vi "RT main 2 local variable.vi"() -> ()   [LabVIEW 2017]
doc: "This example demonstrates how to acquire a continuous amount of data (Waveform) using the DAQ device's internal clock. It also shows how to synchronize two devices for different device families (E Series, S Series, M Series, X Series, DSA, and SC Express), to simultaneously acquire the data.\n\nFor instructions on how to connect your signals to the DAQ device, refer to your device documentation."
uses:
  typedefs/Data.ctl
  <vilib>/Utility/RT CPU Load.ctl
  <vilib>/Utility/error.llb/DialogType.ctl
  <vilib>/DAQmx/read.llb/DAQmx Read (Analog 1D Wfm NChan NSamp).vi
  <vilib>/Analysis/baseanly.llb/Mean (DBL).vi
  <vilib>/DAQmx/read.llb/DAQmx Read (Analog Wfm 1Chan NSamp).vi
  <vilib>/Analysis/5stat.llb/RMS (DBL).vi
  <vilib>/DAQmx/read.llb/DAQmx Read (Analog DBL 1Chan 1Samp).vi
  <vilib>/DAQmx/create/channels.llb/DAQmx Create Channel (AI-Voltage-Basic).vi
  <vilib>/DAQmx/create/channels.llb/DAQmx Create Channel (AI-Temperature-Thermocouple).vi
  <vilib>/DAQmx/configure/timing.llb/DAQmx Timing (Sample Clock).vi
  <vilib>/httpClient/POSTBuffer.vi
  <vilib>/DAQmx/miscellaneous.llb/DAQmx Fill In Error Info.vi
  <vilib>/Analysis/NI_AALBase.lvlib
  <vilib>/httpClient/LabVIEWHTTPClient.lvlib
  <vilib>/NI_Real-Time Target Support.lvlib
  <vilib>/Analysis/NI_AALPro.lvlib
panel:
  out "output cluster":T1={"RMS"=0.00029761559443340104, "RPM"=4.976174049057853, "Voltage"=24.13586620003172, "Current"=-0.01197022918749992, "Temperature"=22.47037779695891} {"RMS" format="%0.6f"; "RPM" format="%0.2f"; "Voltage" format="%0.2f"; "Current" format="%0.2f"; "Temperature" format="%0.2f"}
  in  "Ipad 1":bool
  in  "Ipad 3":bool
  in  "Ipad 2":bool
  in  "Button 3":bool
  in  "Button 2":bool
  in  "Buttoon 1":bool
  in  "String":string="http://10.156.1.111:8001/cRioWebservice/weURL"
  in  "Tab Control":enum32{"Main", "Setup   ", "Debug"}(tab)=enum."Setup   "
  out "Output States":bool[](array[boolean])
  out "From Thingworx":bool[](array[boolean])
  out "Voltage":dbl(graph)=22.47037779695891 caption="Thermocouple waveform"
  out "Current":dbl(graph)=22.47037779695891 caption="Thermocouple waveform"
  out "RPM":dbl(graph)=22.47037779695891 caption="Thermocouple waveform"
  out "Temperature":dbl(graph)=22.47037779695891 caption="Thermocouple waveform"
  out "Vibration":waveform(dbl)(graph)={"t0"=timestamp(3612407740.6938596 s since 1904-01-01), "dt"=3.906249999999998e-05, "Y"=[], "attributes"=variant("NI_ChannelName"=variant(string "Mod1/ai0"), "NI_UnitDescription"=variant(string "Volts"))}
  out "Data":T2
  out "Buttons":bool[](array[boolean])
  in  "stop":bool
  in  "Vibration Sample":i32=25600
  in  "9234 Sample Rate":dbl=25600.0
  in  "9234 Channel":tag="Mod1/ai0"
  in  "9201 Samples to Read":i32=25600
  in  "9201 Sample Rate":dbl=25600.0
  in  "9201 Channel":tag="Mod3/ai0:2"
  in  "CJC Channel":refnum<k21>
  in  "CJC Value":dbl=25.0 format="%0.2f"
  in  "CJC Source":i32(ring)=10116 items=["Built-In"=10200, "Constant Value"=10116, "Channel"=10113]
  in  "Thermocouple Type":i32(ring)=10073 items=["J"=10072, "K"=10073, "N"=10077, "R"=10082, "S"=10085, "T"=10086, "B"=10047, "E"=10055]
  in  "Units":i32(ring)=10143 items=["Deg C"=10143, "Deg F"=10144, "Kelvins"=10325, "Deg R"=10145, "From Custom Scale"=10065]
  in  "Max Temperature":dbl=35.0
  in  "Min Temperature":dbl=-30.0
  in  "Thermocouple Sample":i32=1
  in  "Thermocouple":tag="Mod2/ai0"
  in  "Voltage correction factor":dbl=5.0
  in  "Current correction factor":dbl=10.0
  in  "Thingworx Key":string="1ec2abed-8590-4b69-8e20-7ebb8ff4261c"
  in  "ThingWorx URL":string="http://10.156.1.88:8080/Thingworx/Things/NIMotor/Services/ReceiveData?postParameter=json"
  out "CPU loads":T3[](array[typedef])=[{"Total (%)"=49.32460172385931, "Time Critical (%)"=0.3247606240343923, "Timed Structures (%)"=0.0, "High (%)"=0.0, "Above Normal (%)"=0.0, "Normal (%)"=48.388661684659795, "Background (%)"=0.0, "Idle (%)"=50.67539827614069, "ISR (%)"=0.6111794151651194}, {"Total (%)"=40.05228188925075, "Time Critical (%)"=0.0, "Timed Structures (%)"=0.0, "High (%)"=0.0, "Above Normal (%)"=0.0, "Normal (%)"=39.81026940927922, "Background (%)"=0.0, "Idle (%)"=59.94771811074925, "ISR (%)"=0.24201247997152983}] {"ISR (%)" format="%#.2f"; "Idle (%)" format="%#.2f"; "Background (%)" format="%#.2f"; "Normal (%)" format="%#.2f"; "Above Normal (%)" format="%#.2f"; "High (%)" format="%#.2g"; "Timed Structures (%)" format="%#.2g"; "Time Critical (%)" format="%#.2g"; "Total (%)" format="%#.2g"}
  out "Loop Count":i32=1197
  out "Loop Count 2":i32=1194
  out "Loop Count 3":i32=725
  out "JSON Output":string
  out "error out":errorcluster
  # "(Not Used)"
  # "Vibration"
  # "Motor Voltage"
  # "Motor Current"
  # "RPM"
  # "Temperature"
  # "Thingworx Setup"
  # "9234 Settings"
  # "9201 Settings"
  # "9211 Settings"
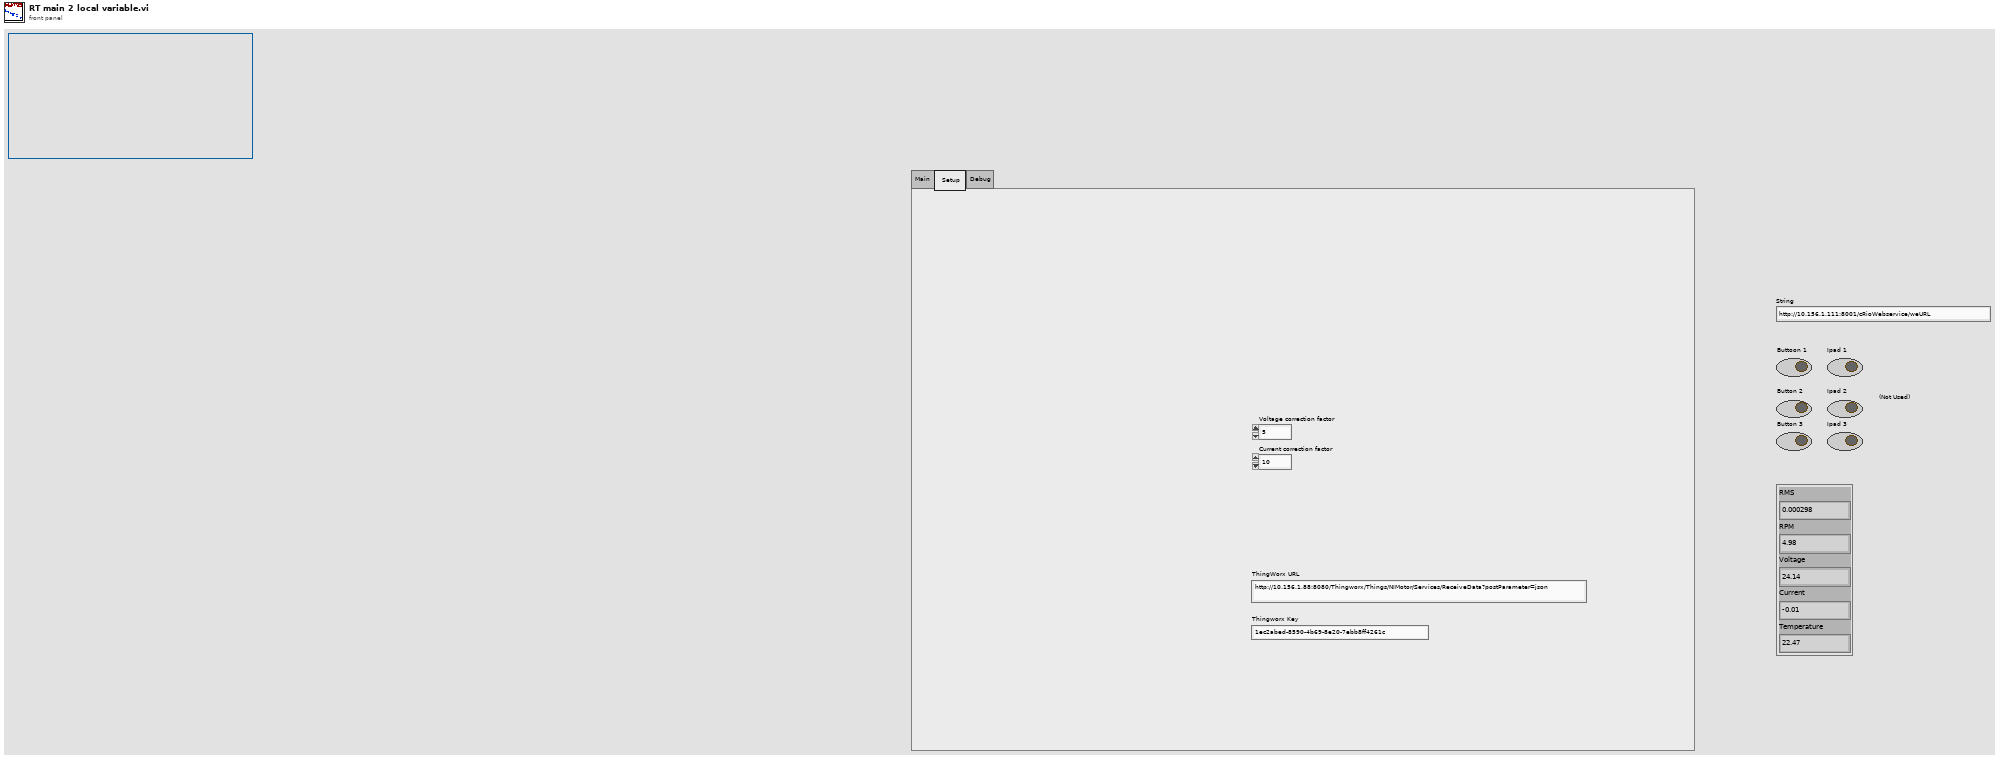
[diagram p1: front panel]
types:
  T1 = typedef "Data.ctl" = cluster{"RMS":dbl, "RPM":dbl, "Voltage":dbl, "Current":dbl, "Temperature":dbl}
  T2 = cluster{"RMS":dbl, "RPM":dbl, "Voltage":dbl, "Current":dbl, "Temperature":dbl}
  T3 = typedef "NI_Real-Time Target Support.lvlib/RT CPU Load.ctl" = cluster{"Total (%)":dbl, "Time Critical (%)":dbl, "Timed Structures (%)":dbl, "High (%)":dbl, "Above Normal (%)":dbl, "Normal (%)":dbl, "Background (%)":dbl, "Idle (%)":dbl, "ISR (%)":dbl}
  T4 = typedef "DialogType.ctl" = u16
  T5 = typedef "LabVIEWHTTPClient.lvlib/ClientHandle.ctl" = refnum<k1>
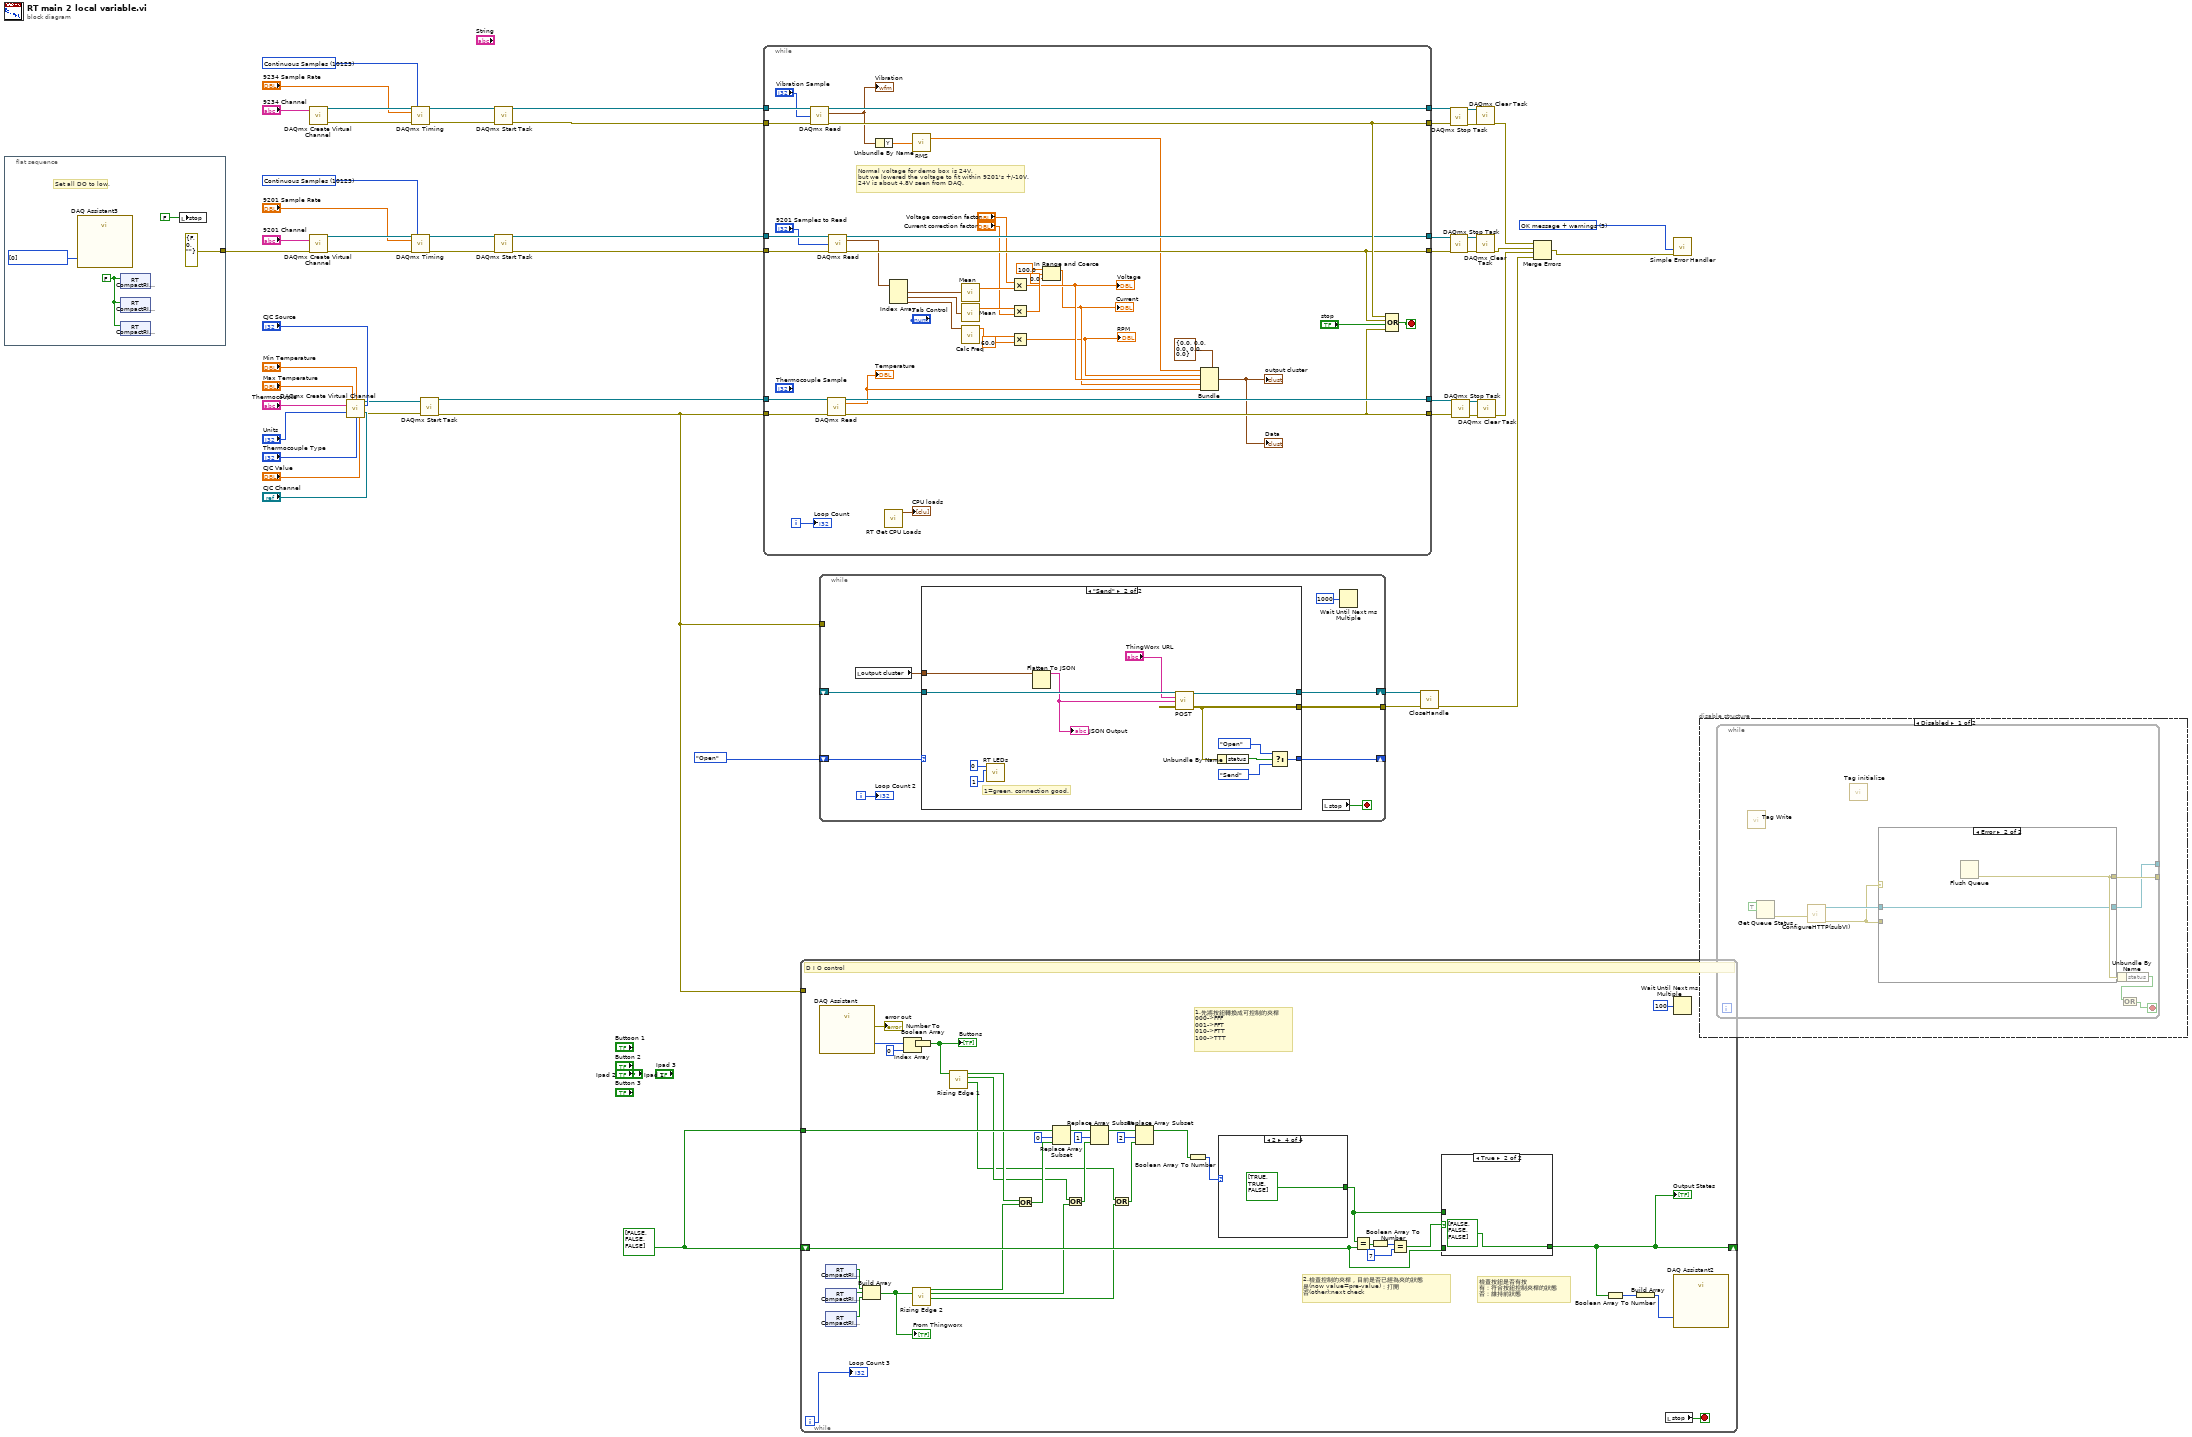
[diagram p0: block diagram]
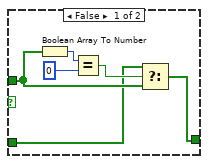
[diagram p2: hidden frame]
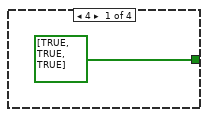
[diagram p3: hidden frame]
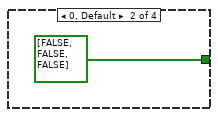
[diagram p4: hidden frame]
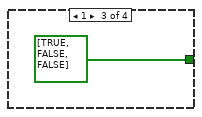
[diagram p5: hidden frame]
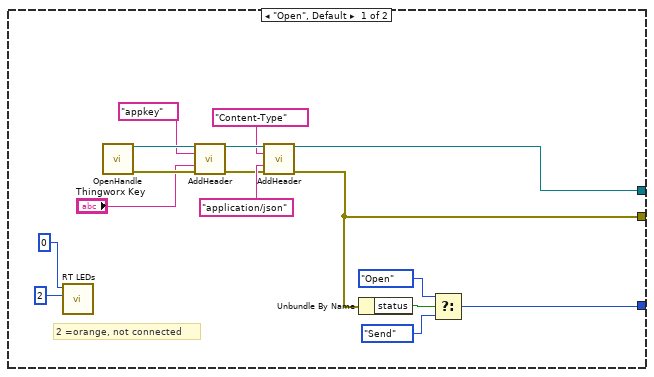
[diagram p6: hidden frame]
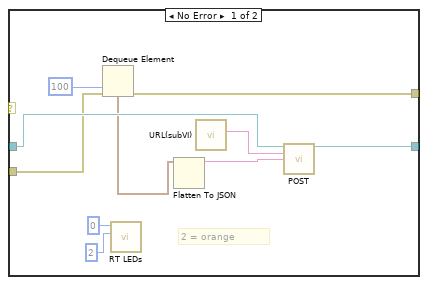
[diagram p7: hidden frame]
diagram:
  w5 = bool[] [FALSE, FALSE, FALSE]
  w10 = 10123 items=["Finite Samples"=10178, "Continuous Samples"=10123, "Hardware Timed Single Point"=12522] ("sample mode")
  w11 = 10123 items=["Finite Samples"=10178, "Continuous Samples"=10123, "Hardware Timed Single Point"=12522] ("sample mode")
  w30 = T4 3 items=["no dialog", "OK message", "continue or stop message", "OK message + warnings", "continue/stop + warnings"] ("type of dialog (OK msg:1)")
  n1 = flat-sequence {
    tunnel: [errorcluster {"status"=FALSE, "code"=0, "source"=""} ("error in")] -> w2
    frame #0 {
      w54 = FALSE ("X")
      # "Set all DO to low."
      n2 = call "DAQ Assistant3"("data"=u32[] [0]) -> ()  [unwired: 17 in, 2 out]
      n3 = shared-variable "RT CompactRIO Target \\variable.lvlib\\X"(w54) -> ()  [unwired: 1 in, 1 out]
      n4 = shared-variable "RT CompactRIO Target \\variable.lvlib\\Y"(w54) -> ()  [unwired: 1 in, 1 out]
      n5 = shared-variable "RT CompactRIO Target \\variable.lvlib\\Z"(w54) -> ()  [unwired: 1 in, 1 out]
      n6 = local write "stop"(FALSE ("Stop")) -> ()
    }
  }
  n7 = call-poly <vilib>:"DAQmx Create Virtual Channel.vi"("physical channels"="9234 Channel") -> ("task out"=w37:refnum<k21>, "error out"=w36:errorcluster)  [unwired: 13 in]
  n8 = call-poly <vilib>:"DAQmx Create Virtual Channel.vi"("physical channels"="9201 Channel", "error in"=w2) -> ("task out"=w33:refnum<k21>, "error out"=w35:errorcluster)  [unwired: 12 in]
  n9 = call-poly <vilib>:"DAQmx Create Virtual Channel.vi"("maximum value"="Max Temperature", "minimum value"="Min Temperature", "physical channels"="Thermocouple", "cjc source"="CJC Source", "units"="Units", "cjc channel"="CJC Channel", "thermocouple type"="Thermocouple Type", "cjc value"="CJC Value") -> ("task out"=w13:refnum<k21>, "error out"=w9:errorcluster)  [unwired: 6 in]
  n10 = call-poly <vilib>:"DAQmx Timing.vi"("task/channels in"=w37, "sample mode"=w10, "rate"="9234 Sample Rate", "error in"=w36) -> ("task out"=w12:refnum<k21>, "error out"=w28:errorcluster)  [unwired: 10 in]
  n11 = call-poly <vilib>:"DAQmx Timing.vi"("task/channels in"=w33, "sample mode"=w11, "rate"="9201 Sample Rate", "error in"=w35) -> ("task out"=w34:refnum<k21>, "error out"=w32:errorcluster)  [unwired: 10 in]
  n12 = call <vilib>:"DAQmx Start Task.vi"("task/channels in"=w13, "error in"=w9) -> ("task out"=w27:refnum<k21>, "error out"=w1:errorcluster)  [unwired: 12 in]
  n13 = call <vilib>:"DAQmx Start Task.vi"("task/channels in"=w12, "error in"=w28) -> ("task out"=w53:refnum<k21>, "error out"=w52:errorcluster)  [unwired: 12 in]
  n14 = call <vilib>:"DAQmx Start Task.vi"("task/channels in"=w34, "error in"=w32) -> ("task out"=w51:refnum<k21>, "error out"=w50:errorcluster)  [unwired: 12 in]
  n15 = while {
    tunnel: w27 -> [w89]
    tunnel: w1 -> [w88]
    tunnel: [w87] -> w24
    tunnel: [w86] -> w23
    tunnel: w53 -> [w96]
    tunnel: [w80] -> w49
    tunnel: w51 -> [w93]
    tunnel: [w81] -> w45
    tunnel: w50 -> [w92]
    tunnel: [w91] -> w44
    tunnel: w52 -> [w95]
    tunnel: [w94] -> w48
    i -> [w79]
    stop <- w97 stop-if-true
    # "Normal voltage for demo box is 24V,\nbut we lowered the voltage to fit within 9201's +/-10V.\n24V is about 4.8V seen from DAQ."
    n16 = call-poly <vilib>:"DAQmx Read.vi"("task/channels in"=w96, "number of samples per channel"="Vibration Sample", "error in"=w95) -> ("task out"=w80:refnum<k21>, "data"=w77:waveform(dbl), "error out"=w94:errorcluster)  [unwired: 10 in]
    "Vibration" <- w77
    n17 = call-poly <vilib>:"DAQmx Read.vi"("task/channels in"=w89, "error in"=w88) -> ("task out"=w87:refnum<k21>, "data"=w83:dbl, "error out"=w86:errorcluster)  [unwired: 11 in]
    "Temperature" <- w83
    n18 = call-poly <vilib>:"DAQmx Read.vi"("task/channels in"=w93, "number of samples per channel"="9201 Samples to Read", "error in"=w92) -> ("task out"=w81:refnum<k21>, "data"=w73:waveform(dbl)[], "error out"=w91:errorcluster)  [unwired: 10 in]
    n19 = Unbundle By Name(w77) -> ("Y"=w76:dbl[])
    n20 = call <vilib>:"RT Get CPU Loads.vi"() -> ("CPU loads"=→"CPU loads":T3[])  [unwired: 10 in, 1 out]
    n21 = Index Array(array=w73) -> (element #1=w84:waveform(dbl), element #2=w82:waveform(dbl), element #3=w68:waveform(dbl))  [unwired: 3 in]
    n22 = call-poly <vilib>:"RMS.vi"("X"=w76) -> ("rms value"=w75:dbl)  [unwired: 1 out]
    n23 = call-poly <vilib>:"Mean.vi"("X"=w82) -> ("mean"=w70:dbl)  [unwired: 1 out]
    n24 = call "Calc Freq.vi"("waveform"=w68) -> ("Freq"=w67:dbl)  [unwired: 10 in]
    n25 = call-poly <vilib>:"Mean.vi"("X"=w84) -> ("mean"=w72:dbl)  [unwired: 1 out]
    n26 = Multiply(x="Voltage correction factor", y=w72) -> (x*y=w62:dbl)
    "Voltage" <- w62
    n27 = Multiply(x=w70, y="Current correction factor") -> (x*y=w65:dbl)
    n28 = Multiply(x=w67, y=60.0) -> (x*y=w60:dbl)
    "RPM" <- w60
    n29 = In Range and Coerce(upper limit=100.0, x=w65, lower limit=0.0) -> (coerced(x)=w61:dbl)  [unwired: 1 out]
    "Current" <- w61
    n30 = Bundle(cluster=T1 {"RMS"=0.0, "RPM"=0.0, "Voltage"=0.0, "Current"=0.0, "Temperature"=0.0} ("Data"), "RMS"=w75, "RPM"=w60, "Voltage"=w62, "Current"=w61, "Temperature"=w83) -> (→"output cluster" →"Data":T1)
    n31 = Compound Arithmetic op=OR(w94, w91, "stop", w86) -> (w97:bool)
    "Loop Count" <- w79
  }
  n32 = while {
    shift-right: [w98] -> _
    shift-left: w5 -> [w119]
    tunnel: w5 -> [w118]
    tunnel: w1 -> [_]
    i -> [w110]
    stop <- w117 stop-if-true
    # "1.先將按鈕轉換成可控制的夾桿\n000->FFF\n001->FFT\n010->FTT\n100->TTT"
    # "檢查按鈕是否有按\n有：符合按鈕控制夾桿的狀態\n否：維持前狀態"
    # "2.檢查控制的夾桿，目前是否已經為夾的狀態\n是(now value=pre-value)：打開\n否(other):next check"
    # "D I O control"
    n33 = call "DAQ Assistant"() -> ("data"=w116:u32[], "error out"=→"error out":errorcluster)  [unwired: 17 in, 1 out]
    n34 = shared-variable "RT CompactRIO Target \\variable.lvlib\\X"() -> (w106:bool)  [unwired: 1 in, 1 out]
    n35 = shared-variable "RT CompactRIO Target \\variable.lvlib\\Y"() -> (w105:bool)  [unwired: 1 in, 1 out]
    n36 = shared-variable "RT CompactRIO Target \\variable.lvlib\\Z"() -> (w104:bool)  [unwired: 1 in, 1 out]
    n37 = Build Array(w106, w105, w104) -> (w99:bool[])
    "From Thingworx" <- w99
    n38 = Index Array(array=w116, index=0) -> (element=w114:u32)
    n39 = call "Rising Edge 2.vi"("Boolean Array"=w99) -> ("triggered? 3"=w101:bool, "triggered? 2"=w102:bool, "triggered? 1"=w103:bool)  [unwired: 8 in]
    n40 = Number To Boolean Array(number=w114) -> (Boolean array=w100:bool[])
    "Buttons" <- w100
    n41 = call "Rising Edge 1.vi"("Boolean Array"=w100) -> ("triggered? 3"=w111:bool, "triggered? 2"=w112:bool, "triggered? 1"=w113:bool)  [unwired: 8 in]
    n42 = Or(x=w113, y=w103) -> (x .or. y?=w129:bool)
    n43 = Replace Array Subset(array=w118, new element=w129, index=0) -> (w134:bool[])
    n44 = Or(x=w112, y=w102) -> (x .or. y?=w128:bool)
    n45 = Replace Array Subset(array=w134, new element=w128, index=1) -> (w133:bool[])
    n46 = Or(x=w111, y=w101) -> (x .or. y?=w127:bool)
    n47 = Replace Array Subset(array=w133, new element=w127, index=2) -> (w120:bool[])
    n48 = Boolean Array To Number(Boolean array=w120) -> (number=w122:u32)
    n49 = case shown="2" w122 {
      tunnel: [bool[] [TRUE, TRUE, TRUE] ("Button") bool[] [FALSE, FALSE, FALSE] ("Button") bool[] [TRUE, FALSE, FALSE] ("Button") bool[] [TRUE, TRUE, FALSE] ("Button")] -> w126
      frame 4 {
      }
      frame 0, Default {
      }
      frame 1 {
      }
      frame 2 {
      }
    }
    n50 = Equal?(x=w126, y=w119) -> (x = y?=w123:bool[])
    n51 = Boolean Array To Number(Boolean array=w123) -> (number=w124:u32)
    n52 = Equal?(x=w124, y=u32 7) -> (x = y?=w125:bool)
    n53 = case shown="True" w125 {
      tunnel: [w136 bool[] [FALSE, FALSE, FALSE] ("Button")] -> w98
      tunnel: w126 -> [w138 _]
      tunnel: w119 -> [w137 _]
      frame False {
        n54 = Boolean Array To Number(Boolean array=w138) -> (number=w140:u32)
        n55 = Equal?(x=w140, y=u32 0) -> (x = y?=w139:bool)
        n56 = Select(t=w137, s=w139, f=w138) -> (s? t:f=w136:bool[])
      }
      frame True {
      }
    }
    "Output States" <- w98
    n57 = Boolean Array To Number(Boolean array=w98) -> (number=w108:u32)
    n58 = Build Array(w108) -> (w107:u32[])
    n59 = local read "stop"() -> (w117:bool)
    n60 = Wait Until Next ms Multiple(millisecond multiple=u32 100) -> ()  [unwired: 1 out]
    n61 = call "DAQ Assistant2"("data"=w107) -> ()  [unwired: 17 in, 2 out]
    "Loop Count 3" <- w110
  }
  n62 = while {
    shift-right: [w154] -> _
    shift-left: enum16{"Open", "Send"}."Open" -> [w155]
    shift-right: [w153] -> w7
    shift-left: _ -> [w152]
    tunnel: [w150] -> w8
    tunnel: w1 -> [_]
    i -> [w149]
    stop <- w151 stop-if-true
    n63 = local read "output cluster"() -> (w147:T1)
    n64 = case shown="\"Send\"" w155 {
      tunnel: [w168 w182] -> w154
      tunnel: [w157 w178] -> w153
      tunnel: w152 -> [_ w179]
      tunnel: [w156 w174] -> w150
      tunnel: w147 -> [_ w173]
      frame "Open", Default {
        # "2 =orange, not connected"
        n65 = call <vilib>:"RT LEDs.vi"("State"=2, "LED Num"=0) -> ()  [unwired: 4 in, 2 out]
        n66 = call <vilib>:"OpenHandle.vi"() -> ("client handle out"=w165:T5, "error out"=w164:errorcluster)  [unwired: 14 in]
        n67 = call <vilib>:"AddHeader.vi"("client handle"=w165, "header"="appkey", "value"="Thingworx Key", "error in (no error)"=w164) -> ("client handle out"=w163:T5, "error out"=w160:errorcluster)  [unwired: 10 in]
        n68 = call <vilib>:"AddHeader.vi"("client handle"=w163, "header"="Content-Type", "value"="application/json", "error in (no error)"=w160) -> ("client handle out"=w157:T5, "error out"=w156:errorcluster)  [unwired: 10 in]
        n69 = Unbundle By Name(w156) -> ("status"=w171:bool)
        n70 = Select(t=enum16{"Open", "Send"}."Open", s=w171, f=enum16{"Open", "Send"}."Send") -> (s? t:f=w168:enum16{"Open", "Send"})
      }
      frame "Send" {
        # "1=green, connection good."
        n71 = call <vilib>:"RT LEDs.vi"("State"=1, "LED Num"=0) -> ()  [unwired: 4 in, 2 out]
        n72 = Flatten To JSON(anything=w173) -> (JSON string=w175:string)  [unwired: 2 in, 1 out]
        "JSON Output" <- w175
        n73 = call-poly <vilib>:"POST.vi"("client handle"=w179, "url"="ThingWorx URL", "buffer"=w175) -> ("client handle out"=w178:T5, "error out"=w174:errorcluster)  [unwired: 9 in, 2 out]
        n74 = Unbundle By Name(w174) -> ("status"=w183:bool)
        n75 = Select(t=enum16{"Open", "Send"}."Open", s=w183, f=enum16{"Open", "Send"}."Send") -> (s? t:f=w182:enum16{"Open", "Send"})
      }
    }
    n76 = local read "stop"() -> (w151:bool)
    n77 = Wait Until Next ms Multiple(millisecond multiple=u32 1000) -> ()  [unwired: 1 out]
    "Loop Count 2" <- w149
  }
  n78 = call <vilib>:"CloseHandle.vi"("client handle"=w7, "error in (no error)"=w8) -> ("error out"=w3:errorcluster)  [unwired: 13 in]
  n79 = call <vilib>:"DAQmx Stop Task.vi"("task/channels in"=w49, "error in"=w48) -> ("task out"=w46:refnum<k21>, "error out"=w47:errorcluster)  [unwired: 12 in]
  n80 = call <vilib>:"DAQmx Stop Task.vi"("task/channels in"=w45, "error in"=w44) -> ("task out"=w42:refnum<k21>, "error out"=w43:errorcluster)  [unwired: 12 in]
  n81 = call <vilib>:"DAQmx Stop Task.vi"("task/channels in"=w24, "error in"=w23) -> ("task out"=w26:refnum<k21>, "error out"=w25:errorcluster)  [unwired: 12 in]
  n82 = call <vilib>:"DAQmx Clear Task.vi"("task in"=w46, "error in"=w47) -> ("error out"=w41:errorcluster)  [unwired: 13 in]
  n83 = call <vilib>:"DAQmx Clear Task.vi"("task in"=w42, "error in"=w43) -> ("error out"=w40:errorcluster)  [unwired: 13 in]
  n84 = call <vilib>:"DAQmx Clear Task.vi"("task in"=w26, "error in"=w25) -> ("error out"=w22:errorcluster)  [unwired: 13 in]
  n85 = Merge Errors(w41, w40, w22, w3) -> (w4:errorcluster)
  n86 = call <vilib>:"Simple Error Handler.vi"("type of dialog (OK msg:1)"=w30, "error in (no error)"=w4) -> ()  [unwired: 3 in, 5 out]
  n87 = disable-structure shown="Disabled" {
    frame Disabled {
      n88 = while {
        tunnel: [w189] -> _
        tunnel: [w186] -> _
        stop <- w190 stop-if-true
        n89 = call "Tag Write.vi"() -> ()  [unwired: 19 in, 1 out]
        n90 = Get Queue Status(return elements? (F)=TRUE) -> (error out=w188:errorcluster)  [unwired: 2 in, 7 out]
        n91 = call "ConfigureHTTP(subVI).vi"("error in (no error)"=w188) -> ("error out"=w184:errorcluster, "Refnum out"=w187:T5)  [unwired: 9 in]
        n92 = call "Tag initialize.vi"() -> ()  [unwired: 14 in, 6 out]
        n93 = case shown="Error" w184 {
          tunnel: [w197 w203] -> w189
          tunnel: w187 -> [w199 w202]
          tunnel: [w198 w202] -> w186
          tunnel: w184 -> [w196 _]
          frame No Error {
            # "2 = orange"
            n94 = Dequeue Element(timeout in ms (-1)=100, error in (no error)=w196) -> (element=w194:T2, error out=w197:errorcluster)  [unwired: 1 in, 2 out]
            n95 = call <vilib>:"RT LEDs.vi"("State"=2, "LED Num"=0) -> ()  [unwired: 4 in, 2 out]
            n96 = Flatten To JSON(anything=w194) -> (JSON string=w195:string)  [unwired: 2 in, 1 out]
            n97 = call "URL(subVI).vi"() -> ("URL"=w200:string)  [unwired: 11 in]
            n98 = call-poly <vilib>:"POST.vi"("client handle"=w199, "url"=w200, "buffer"=w195) -> ("client handle out"=w198:T5)  [unwired: 9 in, 3 out]
          }
          frame Error {
            n99 = Flush Queue() -> (error out=w203:errorcluster)  [unwired: 2 in, 2 out]
          }
        }
        n100 = Unbundle By Name(w189) -> ("status"=w191:bool)
        n101 = Or(x=w191) -> (x .or. y?=w190:bool)  [unwired: 1 in]
      }
    }
    frame Enabled {
    }
  }
